vi "Config Math.vi"(0 "VISA resource name":refnum<visa-resource-name>, 1 "Element (1: Element 1)":u16(ring)=1 items=["", "Element1", "Element2", "Element3", "Sigma"], 5 "Math Type (0: Crest Factor)":u16(ring) items=["C Factor", "Arithmetic", "Average", "Efficiency"], 7 "C Factor (0: V)":u16(ring) items=["V1", "A1", "V2", "A2", "V3", "A3"], 9 "Arithmetic (0: ADD)":u16(ring) items=["ADD", "SUB", "MUL", "DIV", "DIVA", "DIVB"], 11 "error in (no error)":errorcluster) -> (4 "VISA resource name out":refnum<visa-resource-name>, 15 "error out":errorcluster)   [LabVIEW 2018, in "Yokogawa WT200 Series.lvlib"]
doc: "This VI sends the Math command to the WT200 Series."
uses:
  Yokogawa WT200 Series.lvlib
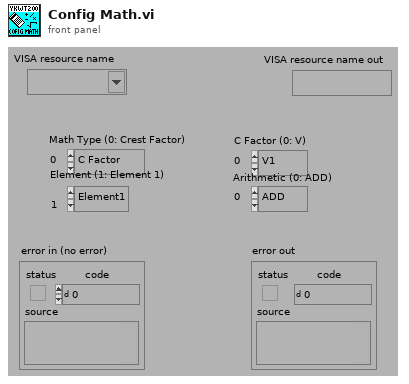
[diagram p1: front panel]
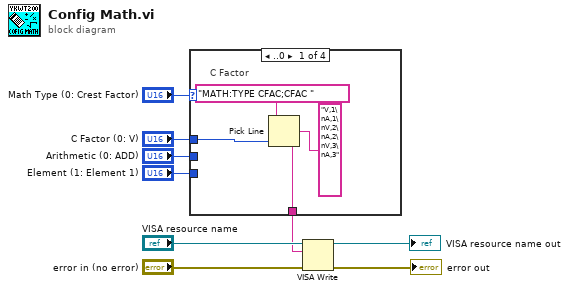
[diagram p0: block diagram]
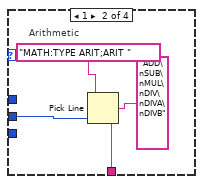
[diagram p2: hidden frame]
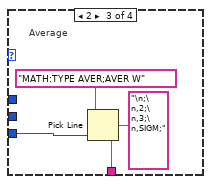
[diagram p3: hidden frame]
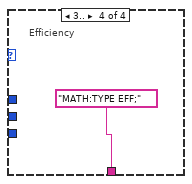
[diagram p4: hidden frame]
diagram:
  n1 = case shown="..0" "Math Type (0: Crest Factor)" {
    tunnel: "Arithmetic (0: ADD)" -> [_ w15 _ _]
    tunnel: [w11 w14 w21 "MATH:TYPE EFF;"] -> w2
    tunnel: "C Factor (0: V)" -> [w10 _ _ _]
    tunnel: "Element (1: Element 1)" -> [_ _ w20 _]
    frame ..0 {
      # "C Factor"
      n2 = Pick Line(string ("")="MATH:TYPE CFAC;CFAC ", multi-line string="V,1\nA,1\nV,2\nA,2\nV,3\nA,3", line index=w10) -> (output string=w11:string)
    }
    frame 1 {
      # "Arithmetic"
      n3 = Pick Line(string ("")="MATH:TYPE ARIT;ARIT ", multi-line string="ADD\nSUB\nMUL\nDIV\nDIVA\nDIVB", line index=w15) -> (output string=w14:string)
    }
    frame 2 {
      # "Average"
      n4 = Pick Line(string ("")="MATH:TYPE AVER;AVER W", multi-line string="\n;\n,2;\n,3;\n,SIGM;" ("ÏÙÁ×²Ý•¶Žš—ñ"), line index=w20) -> (output string=w21:string)
    }
    frame 3.. {
      # "Efficiency"
    }
  }
  n5 = VISA Write(VISA resource name="VISA resource name", write buffer=w2, error in (no error)="error in (no error)") -> (VISA resource name out=→"VISA resource name out":refnum<visa-resource-name>, error out=→"error out":errorcluster)  [unwired: 1 out]
